vi "Stepper Motor.vi"() -> ()   [LabVIEW 2012]
uses:
  <vilib>/DAQmx/create/channels.llb/DAQmx Create Channel (DO-Digital Output).vi
  <vilib>/DAQmx/create/channels.llb/DAQmx Create Channel (AI-Voltage-Basic).vi
  <vilib>/DAQmx/read.llb/DAQmx Read (Analog DBL 1Chan 1Samp).vi
  <vilib>/DAQmx/write.llb/DAQmx Write (Digital U32 1Chan 1Samp).vi
panel:
  in  "lines":tag
  in  "physical channels":tag
  in  "delay":u32
  in  "stop":bool
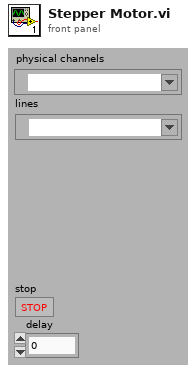
[diagram p1: front panel]
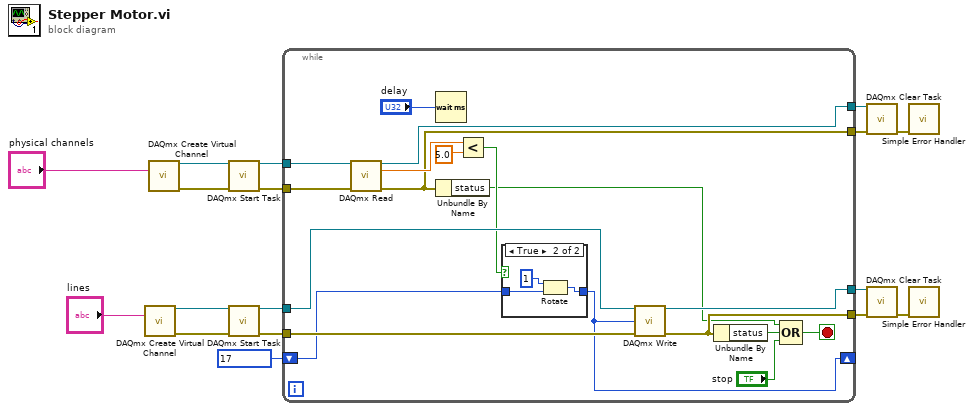
[diagram p0: block diagram]
diagram:
  n1 = call-poly <vilib>:"DAQmx Create Virtual Channel.vi"("lines"="lines") -> ("task out"=w17:refnum<k21>, "error out"=w16:errorcluster)  [unwired: 13 in]
  n2 = call-poly <vilib>:"DAQmx Create Virtual Channel.vi"("physical channels"="physical channels") -> ("task out"=w10:refnum<k21>, "error out"=w11:errorcluster)  [unwired: 13 in]
  n3 = call <vilib>:"DAQmx Start Task.vi"("task/channels in"=w10, "error in"=w11) -> ("task out"=w9:refnum<k21>, "error out"=w8:errorcluster)  [unwired: 12 in]
  n4 = call <vilib>:"DAQmx Start Task.vi"("task/channels in"=w17, "error in"=w16) -> ("task out"=w14:refnum<k21>, "error out"=w15:errorcluster)  [unwired: 12 in]
  n5 = while {
    tunnel: w15 -> [w34]
    tunnel: w14 -> [w35]
    tunnel: [w32] -> w12
    tunnel: [w33] -> w13
    tunnel: w9 -> [w27]
    tunnel: w8 -> [w26]
    tunnel: [w19] -> w5
    tunnel: [w25] -> w6
    shift-right: [w22] -> _
    shift-left: u8 17 -> [w21]
    stop <- w29 stop-if-true
    n6 = call-poly <vilib>:"DAQmx Read.vi"("task/channels in"=w27, "error in"=w26) -> ("task out"=w25:refnum<k21>, "data"=w24:dbl, "error out"=w19:errorcluster)  [unwired: 11 in]
    n7 = Wait (ms)(milliseconds to wait="delay") -> ()  [unwired: 1 out]
    n8 = Unbundle By Name(w19) -> ("status"=w18:bool)
    n9 = Less?(x=w24, y=5.0) -> (x < y?=w20:bool)
    n10 = case shown="True" w20 {
      tunnel: w21 -> [w36 w38]
      tunnel: [w36 w39] -> w22
      frame False {
      }
      frame True {
        n11 = Rotate(1:w38, 2:u8 1 ("x")) -> (0:w39:u8)
      }
    }
    n12 = call-poly <vilib>:"DAQmx Write.vi"("task/channels in"=w35, "data"=w22, "error in"=w34) -> ("task out"=w33:refnum<k21>, "error out"=w32:errorcluster)  [unwired: 10 in, 1 out]
    n13 = Unbundle By Name(w32) -> ("status"=w31:bool)
    n14 = Compound Arithmetic op=OR(w18, w31, "stop") -> (w29:bool)
  }
  n15 = call <vilib>:"DAQmx Clear Task.vi"("task in"=w6, "error in"=w5) -> ("error out"=w4:errorcluster)  [unwired: 13 in]
  n16 = call <vilib>:"DAQmx Clear Task.vi"("task in"=w13, "error in"=w12) -> ("error out"=w3:errorcluster)  [unwired: 13 in]
  n17 = call <vilib>:"Simple Error Handler.vi"("error in (no error)"=w4) -> ()  [unwired: 4 in, 5 out]
  n18 = call <vilib>:"Simple Error Handler.vi"("error in (no error)"=w3) -> ()  [unwired: 4 in, 5 out]
